vi "Configure Event Search (Serial Bus - LIN).vi"(5 "Data Value Format (1: Decimal)":i32(ring)=1 items=["Hex", "Decimal"], 6 "Data Length (4 Bytes)":dbl=4.0, 7 "Data Value (0)":string="0", 8 "error in (no error)":errorcluster, 9 "Frame ID Value (0)":i32, 10 "Search Operation (0: ID)":i32(ring) items=["ID", "Data", "Error"], 11 "VISA resource name":refnum<visa-resource-name>="A") -> (0 "error out":errorcluster, 3 "VISA resource name out":refnum<visa-resource-name>)   [LabVIEW 2010, in "Agilent 2000 3000 X-Series.lvlib"]
doc: "Configures the event search of LIN bus."
uses:
  <instrlib>/Agilent 2000 3000 X-Series/Agilent 2000 3000 X-Series.lvlib
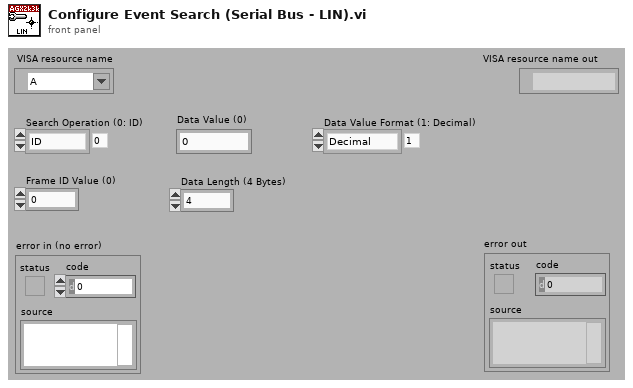
[diagram p1: front panel]
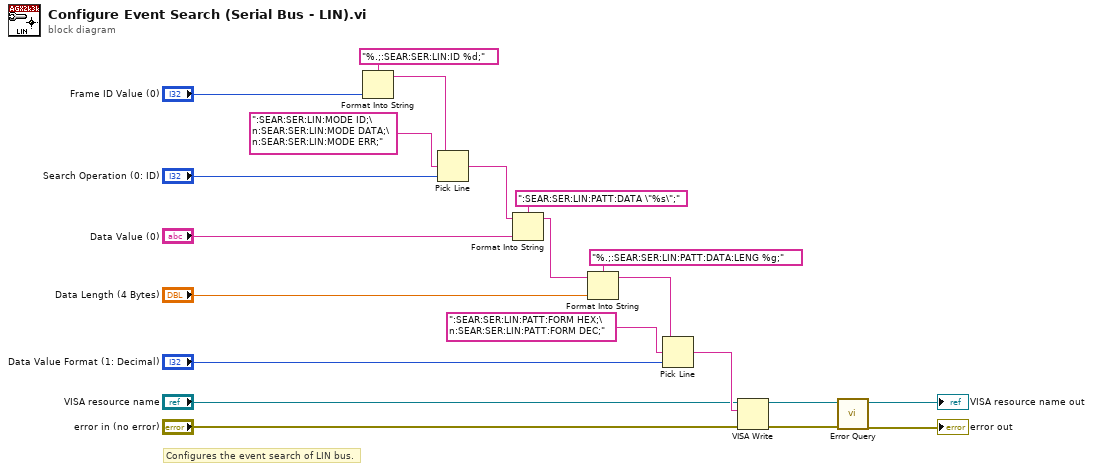
[diagram p0: block diagram]
diagram:
  # "Configures the event search of LIN bus."
  n1 = Format Into String(format string="%.;:SEAR:SER:LIN:ID %d;", "Frame ID Value (0)") -> (resulting string=w17:string)  [unwired: 2 in, 1 out]
  n2 = Pick Line(string ("")=w17, multi-line string=":SEAR:SER:LIN:MODE ID;\n:SEAR:SER:LIN:MODE DATA;\n:SEAR:SER:LIN:MODE ERR;", line index="Search Operation (0: ID)") -> (output string=w16:string)
  n3 = Format Into String(format string=":SEAR:SER:LIN:PATT:DATA \"%s\";", initial string=w16, "Data Value (0)") -> (resulting string=w14:string)  [unwired: 1 in, 1 out]
  n4 = Format Into String(format string="%.;:SEAR:SER:LIN:PATT:DATA:LENG %g;", initial string=w14, "Data Length (4 Bytes)") -> (resulting string=w9:string)  [unwired: 1 in, 1 out]
  n5 = Pick Line(string ("")=w9, multi-line string=":SEAR:SER:LIN:PATT:FORM HEX;\n:SEAR:SER:LIN:PATT:FORM DEC;", line index="Data Value Format (1: Decimal)") -> (output string=w8:string)
  n6 = VISA Write(VISA resource name="VISA resource name", write buffer=w8, error in (no error)="error in (no error)") -> (VISA resource name out=w5:refnum<visa-resource-name>, error out=w4:errorcluster)  [unwired: 1 out]
  n7 = call <instrlib>:"Error Query.vi"("error in (no error)"=w4, "VISA resource name"=w5) -> ("error out"=→"error out":errorcluster, "VISA resource name out"=→"VISA resource name out":refnum<visa-resource-name>)  [unwired: 8 out]
